vi "Set Buttons from Objects.vi"(0 "Display State In":T1={"Buttons Displayed"=0, "Button States"=[], "Button Size"=0, "Button Style"=enum."Classic", "Active Button"=0, "Force Regen?"=FALSE, "Tip String Ref"=refnum}, 5 "Buttons":refnum<class "Button.lvclass">[](array[class]), 7 "Insert (F=Replace)":bool, 9 "Container State":T3, 11 "error in (no error)":errorcluster) -> (4 "Display State Out":T1={"Buttons Displayed"=0, "Button States"=[], "Button Size"=0, "Button Style"=enum."Classic", "Active Button"=0, "Force Regen?"=FALSE, "Tip String Ref"=refnum}, 15 "error out":errorcluster)   [LabVIEW 2018, in "Toolbar.xctl"]
doc: "Set lots of buttons from an array of button class objects in one go."
uses:
  Toolbar.xctl
  <vilib>/_xctls/Container State.ctl
  <vilib>/_xctls/XControlSupport.lvlib
  Button_Class/Button.lvclass
  Toolbar State.ctl
  Button_Class/Type Defs/Button Style.ctl
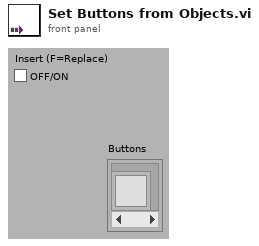
[diagram p1: front panel]
types:
  T1 = typedef "Toolbar.xctl/Toolbar State.ctl" = cluster{"Buttons Displayed":i32, "Button States":refnum<class "Button.lvclass">[], "Button Size":i32, "Button Style":T2, "Active Button":i32, "Force Regen?":bool, "Tip String Ref":refnum<vi>}
  T2 = typedef "Button.lvclass/Button Style.ctl" = enum16{"System", "Modern", "Classic", "Rounded", "Silver", "Ni Theme", "Metallic"}
  T3 = typedef "XControlSupport.lvlib/Container State.ctl" = cluster{"Indicator?":bool, "Run Mode?":bool, " Refnum":refnum<vi>}
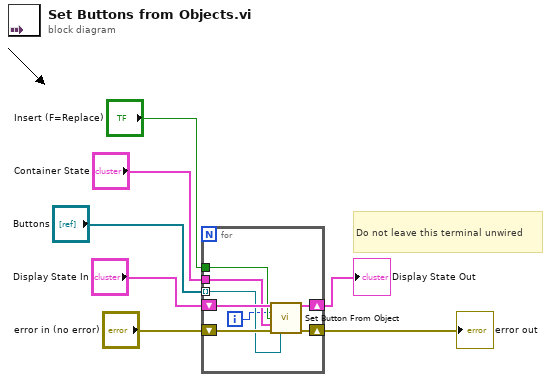
[diagram p0: block diagram]
diagram:
  # "Do not leave this terminal unwired"
  n1 = for {
    shift-right: [w14] -> w1
    shift-left: "Display State In" -> [w15]
    shift-right: [w12] -> w5
    shift-left: "error in (no error)" -> [w13]
    tunnel: "Buttons" -> [w11] mode=indexing
    tunnel: "Container State" -> [w10]
    tunnel: "Insert (F=Replace)" -> [w9]
    i -> [w8]
    n2 = call "Set Button From Object.vi"("Display State In"=w15, "Index (-1=at end)"=w8, "Insert (F=Replace)"=w9, "Container State"=w10, "error in (no error)"=w13, "Button.lvclass"=w11) -> ("Display State Out"=w14:T1, "error out"=w12:errorcluster)  [unwired: 8 out]
  }
  "Display State Out" <- w1
  "error out" <- w5
